vi "Write State.vi"(8 "error in (no error)":errorcluster, 10 "State":enum16{"BallDispPos", "Exit"}(ring), 11 "DispBallTacticVSS in":refnum<class "DispBallTacticVSS.lvclass">) -> (0 "error out":errorcluster, 3 "DispBallTacticVSS out":refnum<class "DispBallTacticVSS.lvclass">)   [LabVIEW 2018, in "DispBallTacticVSS.lvclass"]
uses:
  DispBallTacticVSS.lvclass
  DispBallTacticVSS.lvclass/DispBallTacticVSS.ctl
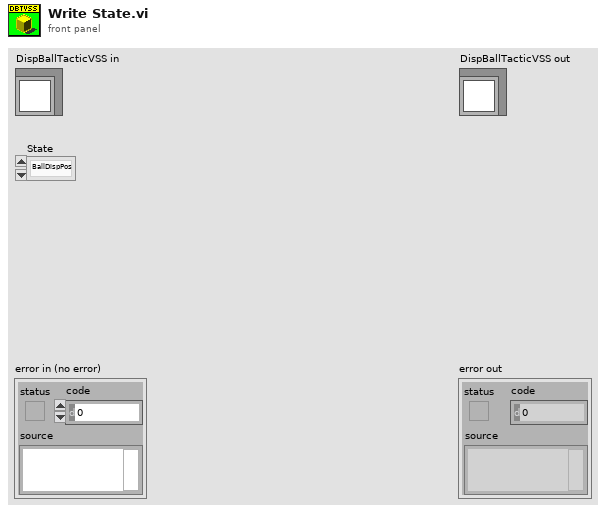
[diagram p1: front panel]
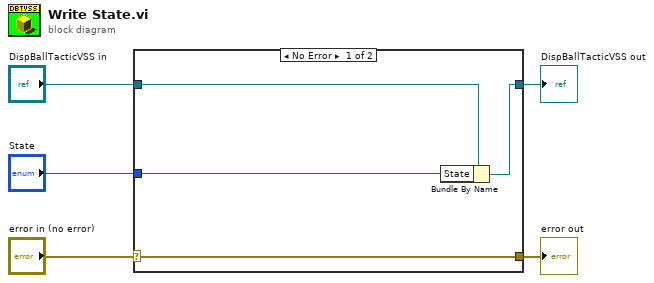
[diagram p0: block diagram]
diagram:
  n1 = case shown="No Error" "error in (no error)" {
    selector: "error in (no error)" -> [w9 w10]
    tunnel: [w9 w10] -> w4
    tunnel: [w7 w11] -> w2
    tunnel: "DispBallTacticVSS in" -> [w8 w11]
    tunnel: "State" -> [w6 _]
    frame No Error {
      n2 = Bundle By Name(cluster=w8, "State"=w6) -> (w7:refnum<class "DispBallTacticVSS.lvclass">)
    }
    frame Error {
    }
  }
  "error out" <- w4
  "DispBallTacticVSS out" <- w2
